vi "Write VISA resource name.vi"(10 "VISA resource name":refnum<visa-resource-name>, 11 "Device in":refnum<class "PIC-Device.lvclass">) -> (3 "Device out":refnum<class "PIC-Device.lvclass">)   [LabVIEW 2020, in "PIC-Device.lvclass"]
uses:
  PIC-Device.lvclass
  PIC-Device.lvclass/PIC-Device.ctl
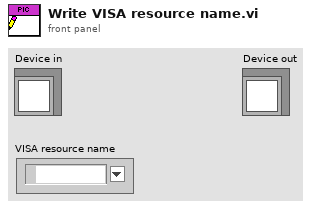
[diagram p1: front panel]
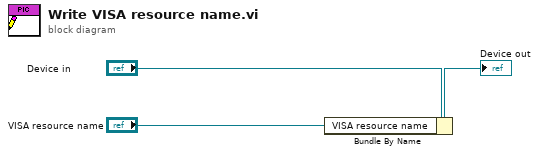
[diagram p0: block diagram]
diagram:
  n1 = Bundle By Name(cluster="Device in", "VISA resource name"="VISA resource name") -> (→"Device out":refnum<class "PIC-Device.lvclass">)
